vi "DIAdem Report Wizard Start CSC.vi"(4 "error in (no error)":errorcluster, 6 "Layout File (Path and File)":path, 7 "Data File (Path and File)":path) -> (0 "error out":errorcluster)   [LabVIEW 2020]
doc: "This VI calls DIAdem to generate a report containing graphs. A Wizard generates the report in DIAdem. Enter the name of the data file for which the report is to be generated as the VI \"Data File\" parameter. The LabVIEW ASCII spreadsheet file format is one of the data formats you can use. If you do not transfer a data file, a dialog for selecting data appears in the Wizard. \n\nDIAdem starts as an independent application. If one or more DIAdem applications are in use when you call the Report Wizard, the VI makes an OLE connection to the last one that was started."
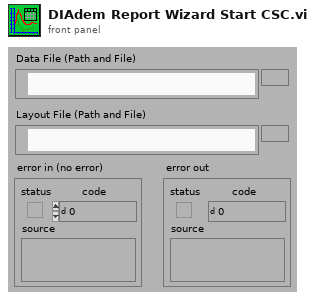
[diagram p1: front panel]
types:
  T1 = typedef "Window Refnum.ctl" = refnum<k1>
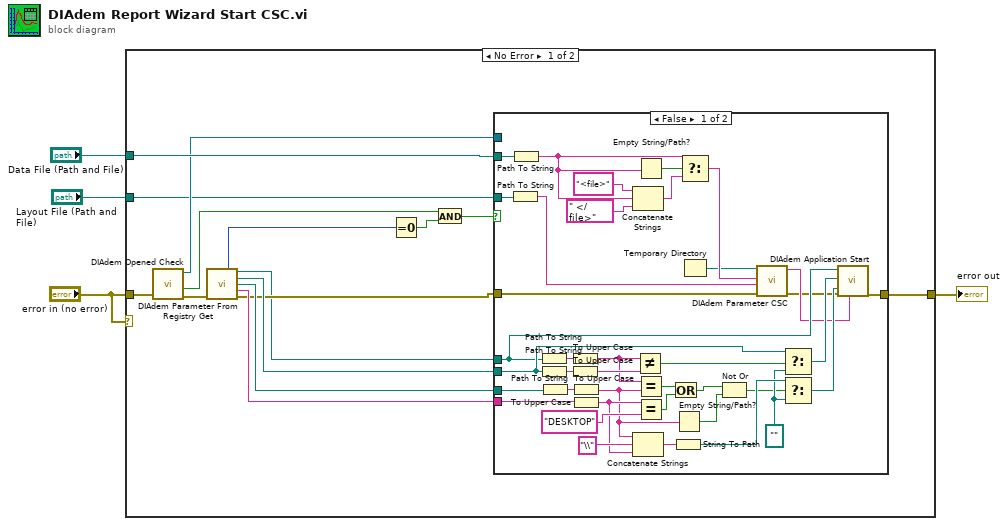
[diagram p0: block diagram]
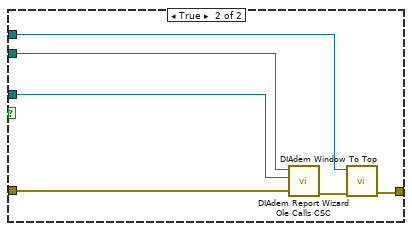
[diagram p2: hidden frame]
diagram:
  n1 = case shown="No Error" "error in (no error)" {
    tunnel: "Data File (Path and File)" -> [w15 _]
    tunnel: [w17 w64] -> w4
    tunnel: "error in (no error)" -> [w18 w64]
    tunnel: "Layout File (Path and File)" -> [w7 _]
    frame No Error {
      n2 = call <vilib>:"DIAdem Opened Check.vi"("error in (no error)"=w18) -> ("DIAdem Window Refnum"=w13:T1, "DIAdem Opened"=w14:bool, "error out"=w12:errorcluster)  [unwired: 1 out]
      n3 = call <vilib>:"DIAdem Parameter From Registry Get.vi"("error in (no error)"=w12) -> ("DIAdem Application Directory"=w5:path, "DIAdem System Directory"=w10:path, "DIAdem Desktop Directory"=w9:path, "DIAdem Desktop File"=w8:string, "DIAdem Instancing Value"=w11:u32, "error out"=w6:errorcluster)  [unwired: 7 in, 2 out]
      n4 = Equal To 0?(x=w11) -> (x = 0?=w16:bool)
      n5 = And(x=w14, y=w16) -> (x .and. y?=w19:bool)
      n6 = case shown="False" w19 {
        tunnel: [w38 w61] -> w17
        tunnel: w15 -> [w36 w63]
        tunnel: w13 -> [_ w60]
        tunnel: w5 -> [w39 _]
        tunnel: w10 -> [w40 _]
        tunnel: w9 -> [w41 _]
        tunnel: w8 -> [w42 _]
        tunnel: w6 -> [w25 w59]
        tunnel: w7 -> [w35 w58]
        frame False {
          w45 = path "" ("f")
          n7 = Path To String(path=w35) -> (string=w26:string)
          n8 = Path To String(path=w36) -> (string=w30:string)
          n9 = Path To String(path=w39) -> (string=w57:string)
          n10 = Path To String(path=w40) -> (string=w56:string)
          n11 = Path To String(path=w41) -> (string=w55:string)
          n12 = To Upper Case(1:w57) -> (0:w53:string)
          n13 = To Upper Case(1:w56) -> (0:w54:string)
          n14 = To Upper Case(1:w55) -> (0:w20:string)
          n15 = To Upper Case(1:w42) -> (0:w49:string)
          n16 = Concatenate Strings("<file>" ("Substring"), w30, " </file>" ("Substring")) -> (w34:string)
          n17 = Concatenate Strings(w20, "\\" ("Substring"), w49) -> (w48:string)
          n18 = Not Equal?(x=w53, y=w54) -> (x != y?=w43:bool)
          n19 = Empty String/Path?(string/path=w30) -> (empty?=w31:bool)
          n20 = Equal?(x=w53, y=w20) -> (x = y?=w46:bool)
          n21 = Equal?(x=w49, y="DESKTOP") -> (x = y?=w52:bool)
          n22 = Or(x=w46, y=w52) -> (x .or. y?=w23:bool)
          n23 = String To Path(string=w48) -> (path=w47:path)
          n24 = Empty String/Path?(string/path=w20) -> (empty?=w22:bool)
          n25 = Select(t=w30, s=w31, f=w34) -> (s? t:f=w27:string)
          n26 = Temporary Directory() -> (w24:path)
          n27 = Not Or(1:w22, 2:w23) -> (0:w21:bool)
          n28 = call <vilib>:"DIAdem Parameter CSC.vi"("error in (no error)"=w25, "Additional Parameter"=w26, "Parameter"=w27, "File Directory"=w24) -> ("error out"=w28:errorcluster, "DIAdem Command Parameter"=w29:string)  [unwired: 2 in]
          n29 = Select(t=w40, s=w43, f=w45) -> (s? t:f=w44:path)
          n30 = Select(t=w47, s=w21, f=w45) -> (s? t:f=w37:path)
          n31 = call <vilib>:"DIAdem Application Start.vi"("DIAdem Additional Start Parameters"=w29, "error in (no error)"=w28, "DIAdem Desktop File"=w37, "DIAdem System Directory"=w44, "DIAdem Directory"=w39) -> ("error out"=w38:errorcluster)  [unwired: 4 in]
        }
        frame True {
          n32 = call <vilib>:"DIAdem Report Wizard Ole Calls CSC.vi"("error in (no error)"=w59, "Layout File (Path and File)"=w58, "Data File (Path and File)"=w63) -> ("error out"=w62:errorcluster)  [unwired: 8 in]
          n33 = call <vilib>:"DIAdem Window To Top.vi"("error in (no error)"=w62, "window refnum"=w60) -> ("error out"=w61:errorcluster)  [unwired: 5 in]
        }
      }
    }
    frame Error {
    }
  }
  "error out" <- w4
